vi "Tree Data Lookup.vi"(10 "Value":string, 11 "Key":string) -> (3 "Tree Data":T1 {"Data Type" items=["Tree Parent"=-1, "Numeric"=0, "String"=1, "Boolean"=2, "Enum"=3]})   [LabVIEW 2020, in "Sequencer with Output Values.lvlib" / "Sequencer with Output Values.lvclass"]
uses:
  Sequencer with Output Values.lvclass
  Tree Item Settings.ctl
  Data Type.ctl
  Global Tree Data.vi
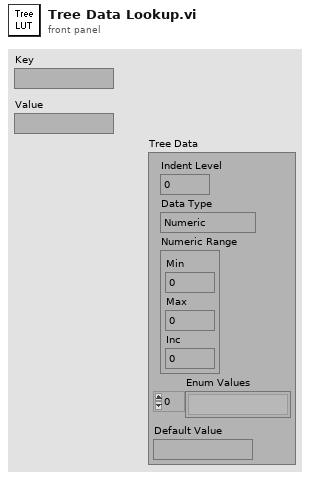
[diagram p1: front panel]
types:
  T1 = typedef "Sequencer with Output Values.lvlib/Sequencer with Output Values.lvclass/Tree Item Settings.ctl" = cluster{"Indent Level":i32, "Data Type":T2, "Numeric Range":cluster{"Min":dbl, "Max":dbl, "Inc":dbl}, "Enum Values":string[], "Default Value":string}
  T2 = typedef "Sequencer with Output Values.lvlib/Sequencer with Output Values.lvclass/Data Type.ctl" = i16
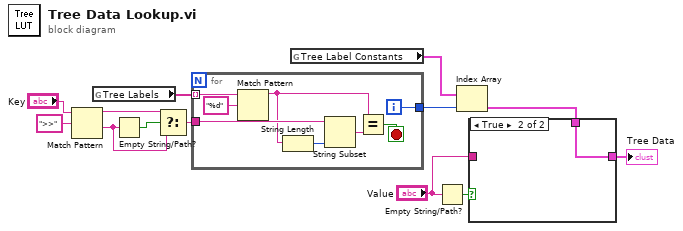
[diagram p0: block diagram]
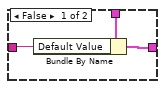
[diagram p2: hidden frame]
diagram:
  n1 = Match Pattern(string="Key", regular expression=">>") -> (before substring=w4:string, after substring=w2:string)  [unwired: 1 in, 2 out]
  n2 = global read "Global Tree Data.vi" "Tree Labels"() -> (w8:string[])
  n3 = Empty String/Path?(string/path=w2) -> (empty?=w3:bool)
  n4 = Select(t=w4, s=w3, f=w2) -> (s? t:f=w1:string)
  n5 = for {
    tunnel: w8 -> [w21] mode=indexing
    tunnel: w1 -> [w19]
    tunnel: [w14] -> w7
    i -> [w14]
    stop <- w15 stop-if-true
    n6 = Match Pattern(string=w21, regular expression="%d") -> (before substring=w17:string)  [unwired: 1 in, 3 out]
    n7 = String Length(string=w17) -> (length=w18:i32)
    n8 = String Subset(string=w19, length (rest)=w18) -> (substring=w16:string)  [unwired: 1 in]
    n9 = Equal?(x=w17, y=w16) -> (x = y?=w15:bool)
  }
  n10 = global read "Global Tree Data.vi" "Tree Label Constants"() -> (w9:T1[])
  n11 = Empty String/Path?(string/path="Value") -> (empty?=w11:bool)
  n12 = Index Array(array=w9, index=w7) -> (element=w13:T1)
  n13 = case shown="True" w11 {
    tunnel: w13 -> [w24 w25]
    tunnel: [w23 w25] -> w10
    tunnel: "Value" -> [w22 _]
    frame False {
      n14 = Bundle By Name(cluster=w24, "Default Value"=w22) -> (w23:T1)
    }
    frame True {
    }
  }
  "Tree Data" <- w10
